vi "_replaceFileExt.vi"(10 "file extensions":string[](array[string]), 11 "path":path) -> (2 "matchPattern":string, 3 "path out":path)   [LabVIEW 2017]
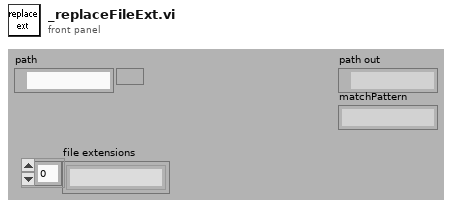
[diagram p1: front panel]
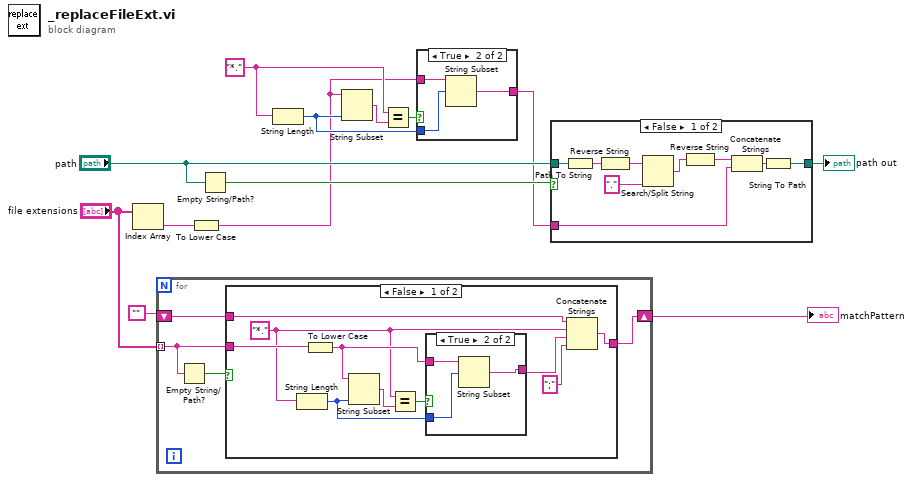
[diagram p0: block diagram]
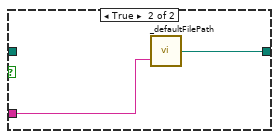
[diagram p5: hidden frame]
diagram:
  w4 = "*." ("string")
  n1 = Index Array(array="file extensions") -> (element=w10:string)  [unwired: 1 in]
  n2 = for {
    tunnel: "file extensions" -> [w15] mode=indexing
    shift-right: [w17] -> w7
    shift-left: "" -> [w16]
    n3 = Empty String/Path?(string/path=w15) -> (empty?=w14:bool)
    n4 = case shown="False" w14 {
      tunnel: w15 -> [w27 _]
      tunnel: [w20 w32] -> w17
      tunnel: w16 -> [w21 w32]
      frame False {
        w19 = "*." ("string")
        n5 = String Length(string=w19) -> (length=w18:i32)
        n6 = To Lower Case(string=w27) -> (all lower case string=w22:string)
        n7 = String Subset(string=w22, length (rest)=w18) -> (substring=w23:string)  [unwired: 1 in]
        n8 = Equal?(x=w19, y=w23) -> (x = y?=w24:bool)
        n9 = case shown="True" w24 {
          tunnel: [w28 w29] -> w26
          tunnel: w22 -> [w28 w31]
          tunnel: w18 -> [_ w30]
          frame False {
          }
          frame True {
            n10 = String Subset(string=w31, offset (0)=w30) -> (substring=w29:string)  [unwired: 1 in]
          }
        }
        n11 = Concatenate Strings(w21, w19, w26, ";" ("string")) -> (w20:string)
      }
      frame True {
      }
    }
  }
  "matchPattern" <- w7
  n12 = To Lower Case(string=w10) -> (all lower case string=w2:string)
  n13 = Empty String/Path?(string/path="path") -> (empty?=w11:bool)
  n14 = String Length(string=w4) -> (length=w3:i32)
  n15 = String Subset(string=w2, length (rest)=w3) -> (substring=w5:string)  [unwired: 1 in]
  n16 = Equal?(x=w4, y=w5) -> (x = y?=w6:bool)
  n17 = case shown="True" w6 {
    tunnel: [w33 w34] -> w1
    tunnel: w2 -> [w33 w36]
    tunnel: w3 -> [_ w35]
    frame False {
    }
    frame True {
      n18 = String Subset(string=w36, offset (0)=w35) -> (substring=w34:string)  [unwired: 1 in]
    }
  }
  n19 = case shown="False" w11 {
    tunnel: [w43 w47] -> w13
    tunnel: w1 -> [w37 w46]
    tunnel: "path" -> [w41 _]
    frame False {
      n20 = Path To String(path=w41) -> (string=w45:string)
      n21 = Reverse String(1:w45) -> (0:w40:string)
      n22 = Search/Split String(string=w40, search string/char (-)=".") -> (match + rest of string=w39:string)  [unwired: 1 in, 2 out]
      n23 = Reverse String(1:w39) -> (0:w38:string)
      n24 = Concatenate Strings(w38, w37) -> (w44:string)
      n25 = String To Path(string=w44) -> (path=w43:path)
    }
    frame True {
      n26 = call <vilib>:"_defaultFilePath.vi"("Storage format"=w46) -> ("File path"=w47:path)  [unwired: 1 in]
    }
  }
  "path out" <- w13
